vi "Save_Log_File(Subvi).vi"(0 "TX_Station":i32, 1 "RX_Station":i32, 3 "1D data":i32[](array[numeric]) caption="1D 데이터") -> (8 "참조 번호 출력":refnum<file>)   [LabVIEW 2023]
uses:
  <vilib>/Utility/sysdir.llb/System Directory Type.ctl
  <vilib>/Utility/file.llb/Write Delimited Spreadsheet (I64).vi
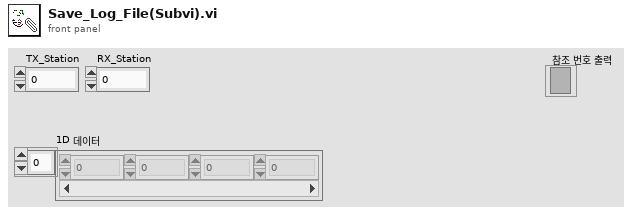
[diagram p1: front panel]
types:
  T1 = enum16{"open", "replace", "create", "open or create", "replace or create", "replace or create with confirmation"}
  T2 = typedef "System Directory Type.ctl" = i32
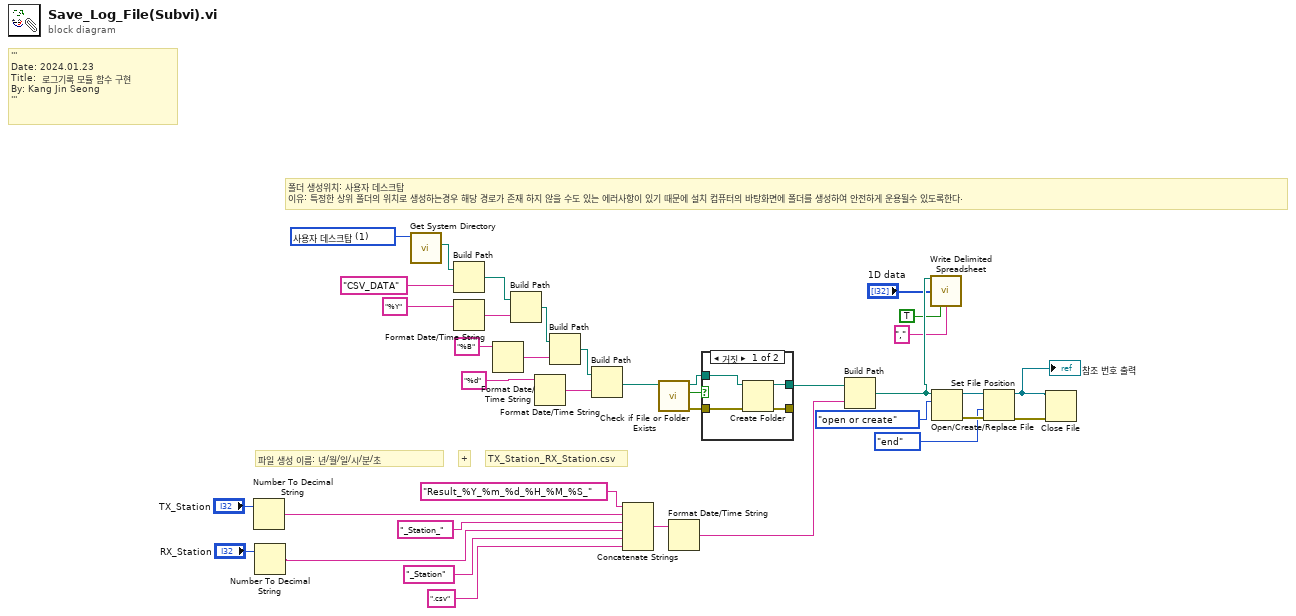
[diagram p0: block diagram]
diagram:
  w31 = T2 1 items=["사용자 홈"=0, "사용자 데스크탑"=1, "사용자 문서"=2, "사용자 어플리케이션 데이터"=3, "사용자 환경"=4, "사용자 임시"=5, "퍼블릭 문서"=6, "퍼블릭 어플리케이션 데이터"=7, "퍼블릭 환경"=8, "퍼블릭 캐시"=13, "시스템 코어 라이브러리"=9, "시스템 설치된 라이브러리"=10, "어플리케이션 파일"=11, "부팅 볼륨 루트"=12] ("system directory type")
  # "+"
  # "TX_Station_RX_Station.csv"
  # "파일 생성 이름: 년/월/일/시/분/초"
  # "폴더 생성위치: 사용자 데스크탑\n이유: 특정한 상위 폴더의 위치로 생성하는경우 해당 경로가 존재 하지 않을 수도 있는 에러사항이 있기 때문에 설치 컴퓨터의 바탕화면에 폴더를 생성하여 안전하게 운용될수 있도록한다."
  # "'''\nDate: 2024.01.23\nTitle:  로그기록 모듈 함수 구현\nBy: Kang Jin Seong\n'''"
  n1 = Number To Decimal String(number="TX_Station") -> (decimal integer string=w6:string)  [unwired: 1 in]
  n2 = Number To Decimal String(number="RX_Station") -> (decimal integer string=w3:string)  [unwired: 1 in]
  n3 = call <vilib>:"Get System Directory.vi"("system directory type"=w31) -> ("system directory"=w37:path)  [unwired: 10 in]
  n4 = Build Path(base path=w37, name or relative path="CSV_DATA") -> (appended path=w25:path)
  n5 = Format Date/Time String(time format string (%c)="%Y") -> (date/time string=w23:string)  [unwired: 2 in]
  n6 = Format Date/Time String(time format string (%c)="%B") -> (date/time string=w22:string)  [unwired: 2 in]
  n7 = Build Path(base path=w25, name or relative path=w23) -> (appended path=w21:path)
  n8 = Format Date/Time String(time format string (%c)="%d") -> (date/time string=w19:string)  [unwired: 2 in]
  n9 = Build Path(base path=w21, name or relative path=w22) -> (appended path=w18:path)
  n10 = Build Path(base path=w18, name or relative path=w19) -> (appended path=w16:path)
  n11 = Concatenate Strings("Result_%Y_%m_%d_%H_%M_%S_" ("시간 포맷 문자열 (%c)"), w6, "_Station_" ("시간 포맷 문자열 (%c)"), w3, "_Station" ("시간 포맷 문자열 (%c)"), ".csv" ("시간 포맷 문자열 (%c)")) -> (w11:string)
  n12 = call <vilib>:"Check if File or Folder Exists.vi"("path"=w16) -> ("error out"=w34:errorcluster, "file or folder exists?"=w36:bool, "dup path"=w35:path)  [unwired: 8 in]
  n13 = Format Date/Time String(time format string (%c)=w11) -> (date/time string=w26:string)  [unwired: 2 in]
  n14 = case shown="거짓" w36 {
    tunnel: w35 -> [w41 w43]
    tunnel: w34 -> [w40 w42]
    tunnel: [w39 w43] -> w27
    tunnel: [w38 w42] -> _
    frame False {
      n15 = Create Folder(path (use dialog)=w41, error in=w40) -> (created path=w39:path, error out=w38:errorcluster)  [unwired: 1 in, 1 out]
    }
    frame True {
    }
  }
  n16 = Build Path(base path=w27, name or relative path=w26) -> (appended path=w10:path)
  n17 = call-poly <vilib>:"Write Delimited Spreadsheet.vi"("file path (dialog if empty)"=w10, "1D data"="1D data", "transpose? (no:F)"=TRUE, "delimiter (\\t)"="," ("delimiter (\\t)")) -> ()  [unwired: 10 in, 2 out]
  n18 = Open/Create/Replace File(file path (use dialog)=w10, operation (0:open)=T1."open or create" ("동작(0:open)")) -> (refnum out=w30:refnum<file>, error out=w29:errorcluster)  [unwired: 4 in, 1 out]
  n19 = Set File Position(refnum=w30, from (0:start)=enum16{"start", "end", "current"}."end" ("위치(0:start)"), error in=w29) -> (refnum out=w1:refnum<file>, error out=w2:errorcluster)  [unwired: 1 in]
  "참조 번호 출력" <- w1
  n20 = Close File(refnum=w1, error in=w2) -> ()  [unwired: 2 out]
